vi "Data handler-Motor Zstack.vi"(4 "Save image":bool, 6 "Single Frame Data":T2, 8 "error in (no error)":errorcluster, 9 "Live graph data queue in":T1, 10 "Logging queue element in":T5={"Imaging Protocol"=enum."Live Imaging", "Number of Trials"=0, "Frame Size"=512, "# Averaged frames"=0, "Dwell time (us)"=0.0, "Index of Z-plane"=0, "Timelapse?"=FALSE, "Logging process is active"=FALSE, "Speed logging enabled"=FALSE, "tdms file ref"=refnum, "path"=path "", "Trial Number"=0, "Expected # points acquired"=FALSE, "Manually stopped"=FALSE, "Last trial"=FALSE, "Ch0 data"=[], "Ch1 data"=[], "Image Time"=[], "Continuous Time"=[], "Points acquired"={"Ch0 last trial"=0, "Ch1 last trial"=0, "All trials"=0}, "HW Timings File"=refnum} {"Frame Size" items=["100X100"=100, "128X128"=128, "200X200"=200, "256X256"=256, "512X512"=512, "1024x1024"=1024, "2048x2048"=2048]; "Dwell time (us)" format="%#.6g"}, 11 "Image array":T3) -> (0 "error out":errorcluster)   [LabVIEW 2017]
uses:
  Typedefs/Logging queue element.ctl
  Typedefs/Imaging Protocols enum.ctl
  Typedefs/Frame Size.ctl
  Typedefs/Acquired points count.ctl
  User Interface/Queue/Live graphs queue/Typedefs/Live imaging queue element.ctl
  <vilib>/vision/Image Controls.llb/IMAQ Image.ctl
  Typedefs/Frame data dual cluster.ctl
  User Interface/Typedefs/Live graph data queue ref.ctl
  Typedefs/Top level VI states.ctl
  Typedefs/Subpanel close request.ctl
  Global Variables/General Globals.vi
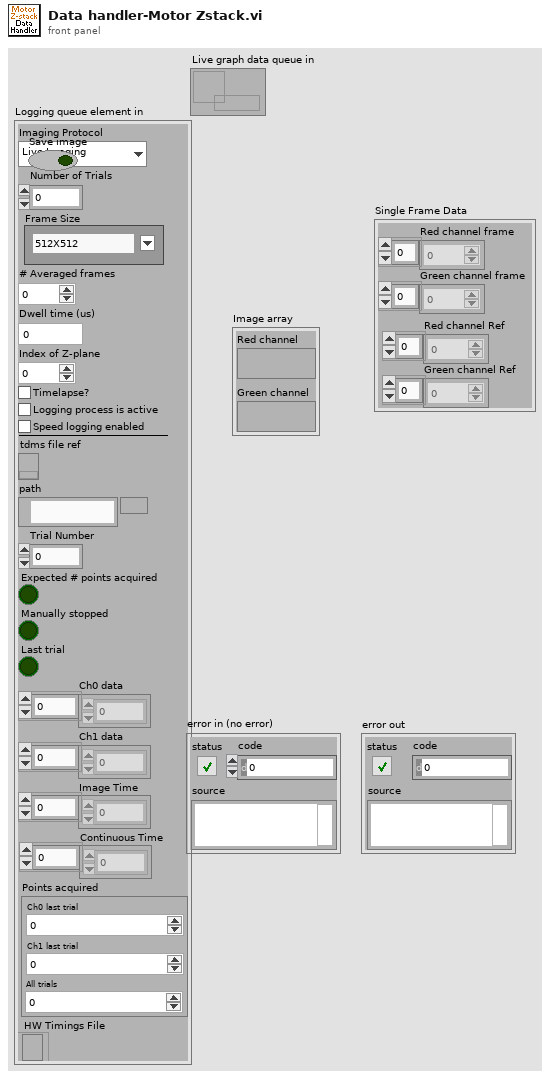
[diagram p1: front panel]
types:
  T1 = typedef "Live graph data queue ref.ctl" = refnum<queue>
  T2 = typedef "Frame data dual cluster.ctl" = cluster{"Red channel frame":dbl[], "Green channel frame":dbl[], "Red channel Ref":dbl[], "Green channel Ref":dbl[]}
  T3 = typedef "Live imaging queue element.ctl" = cluster{"Red channel":T4, "Green channel":T4}
  T4 = typedef "IMAQ Image.ctl" = refnum<image>
  T5 = typedef "Logging queue element.ctl" = cluster{"Imaging Protocol":T6, "Number of Trials":u16, "Frame Size":T7, "# Averaged frames":u16, "Dwell time (us)":dbl, "Index of Z-plane":i32, "Timelapse?":bool, "Logging process is active":bool, "Speed logging enabled":bool, "tdms file ref":refnum<k34>, "path":path, "Trial Number":i32, "Expected # points acquired":bool, "Manually stopped":bool, "Last trial":bool, "Ch0 data":u32[], "Ch1 data":u32[], "Image Time":u64[], "Continuous Time":u64[], "Points acquired":T8, "HW Timings File":refnum<file>}
  T6 = typedef "Imaging Protocols enum.ctl" = enum16{"AOL Z-Stack", "Motor Z Stack", "Functional Acquisition", "Single Plane Acquisition", "Volume Acquisition", "Live Imaging", "Live Plane Imaging", "Live Volume Imaging"}
  T7 = typedef "Frame Size.ctl" = u16
  T8 = typedef "Acquired points count.ctl" = cluster{"Ch0 last trial":u64, "Ch1 last trial":u64, "All trials":u64}
  T9 = typedef "Top level VI states.ctl" = enum16{"None", "Initialise UI", "<STACK PROTOCOL STATES>", "AOL Zstack-START", "AOL Zstack-STOP", "Motor Zstack-START", "Motor Zstack-STOP", "<ACQUISITION PROTOCOL STATES> ", "Functional Acquisition-START", "Functional Acquisition-STOP", "Single Plane Acquisition-START", "Single Plane Acquisition-STOP", "Volume Acquisition-START", "Volume Acquisition-STOP", "<LIVE IMAGING PROTOCOL STATES>", "Live Imaging-START", "Live Imaging-STOP", "Live Plane Imaging-START", "Live Plane Imaging-STOP", "Live Volume Imaging-START", "Live Volume Imaging-STOP", "<MOVEMENT CORRECTION PROTOCOL STATES>", "EXIT"}
  T10 = typedef "Subpanel close request.ctl" = enum16{"Request subpanel close", "Just check subpanel is closed"}
  T11 = enum16{"open", "replace", "create", "open or create", "replace or create", "replace or create with confirmation"}
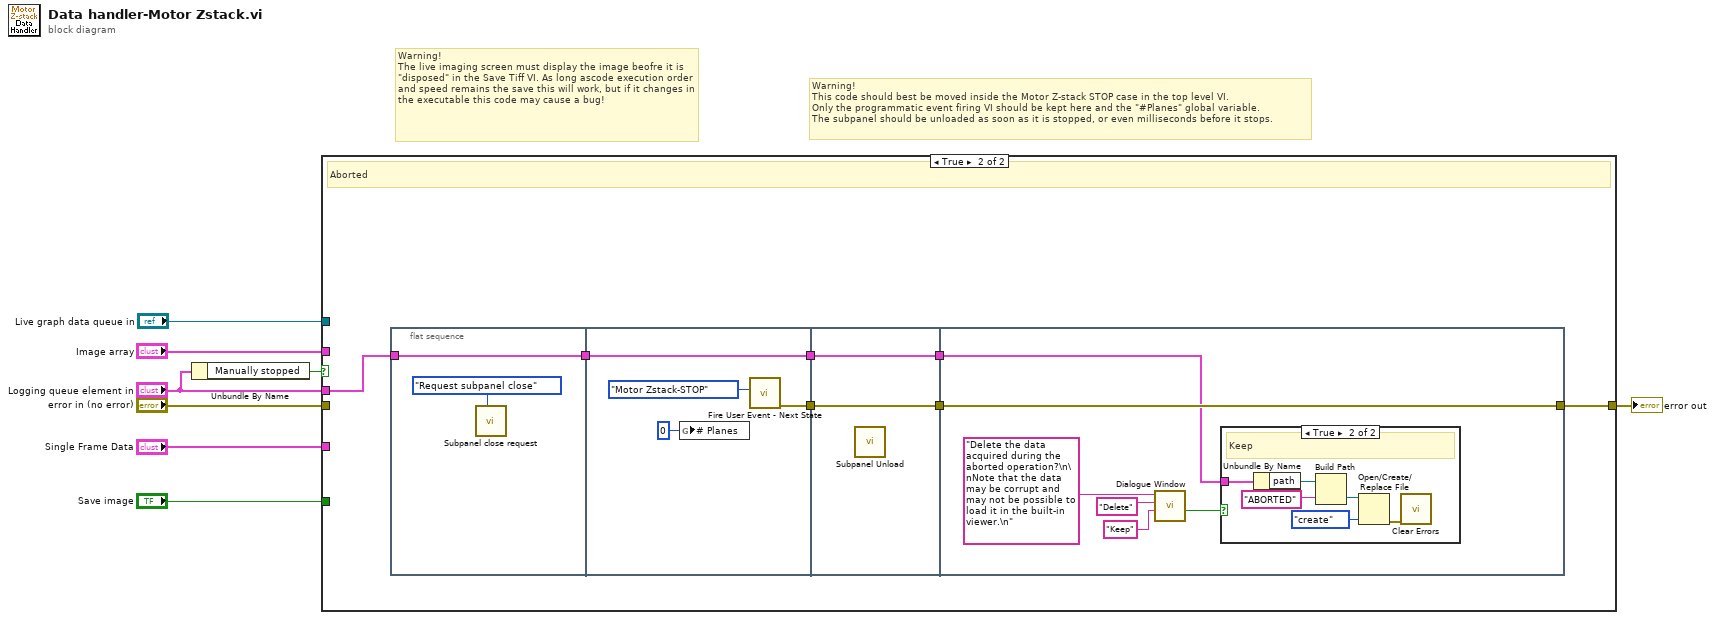
[diagram p0: block diagram]
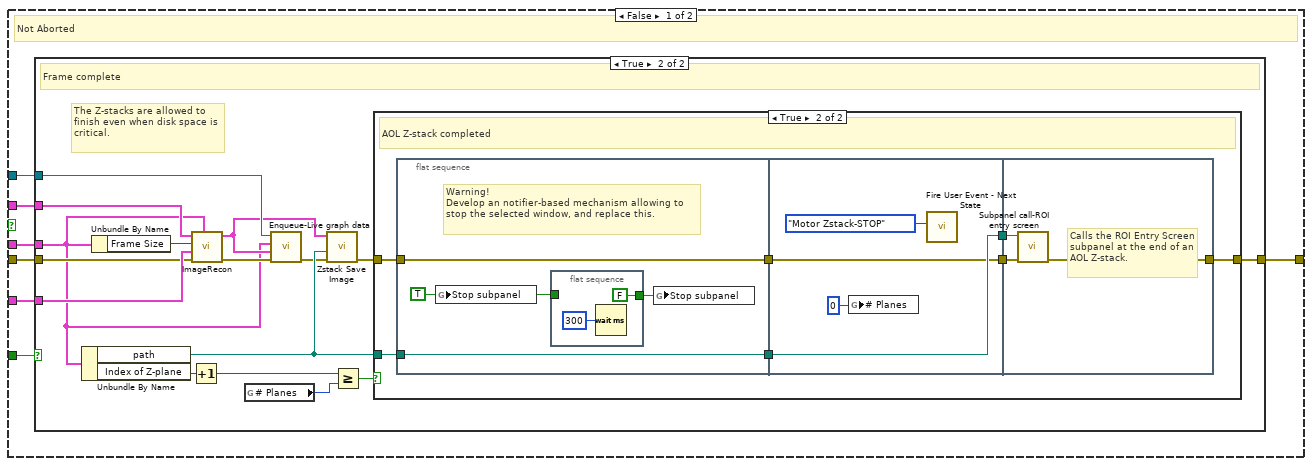
[diagram p2: hidden frame]
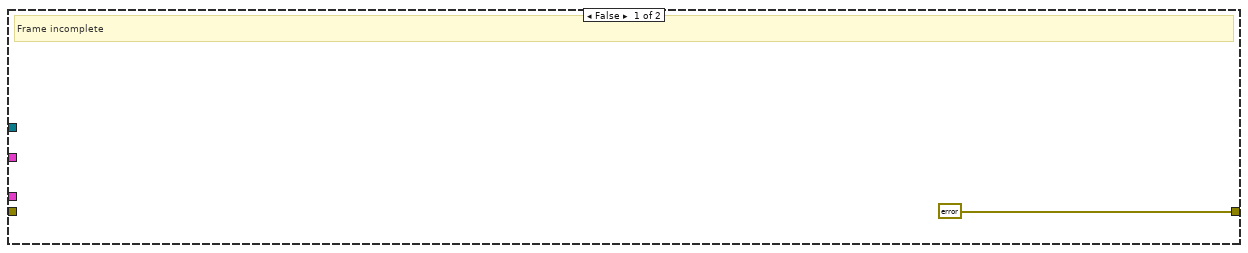
[diagram p3: hidden frame]
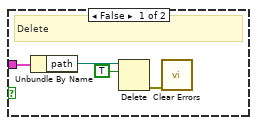
[diagram p5: hidden frame]
diagram:
  # "Warning!\nThe live imaging screen must display the image beofre it is \"disposed\" in the Save Tiff VI. As long ascode execution order and speed remains the save this will work, but if it changes in the executable this code may cause a bug!"
  # "Warning!\nThis code should best be moved inside the Motor Z-stack STOP case in the top level VI.\nOnly the programmatic event firing VI should be kept here and the \"#Planes\" global variable.\nThe subpanel should be unloaded as soon as it is stopped, or even milliseconds before it stops."
  n1 = Unbundle By Name("Logging queue element in") -> ("Manually stopped"=w1:bool)
  n2 = case shown="True" w1 {
    tunnel: [w15 w59] -> w8
    tunnel: "Logging queue element in" -> [w14 w54]
    tunnel: "Image array" -> [w13 _]
    tunnel: "Single Frame Data" -> [w12 _]
    tunnel: "Save image" -> [w11 _]
    tunnel: "error in (no error)" -> [w10 _]
    tunnel: "Live graph data queue in" -> [w9 _]
    frame False {
      # "Not Aborted"
      n3 = case shown="True" w11 {
        tunnel: [errorcluster {"status"=FALSE, "code"=0, "source"=""} ("error out") w32] -> w15
        tunnel: w14 -> [_ w17]
        tunnel: w13 -> [_ w24]
        tunnel: w12 -> [_ w26]
        tunnel: w10 -> [_ w25]
        tunnel: w9 -> [_ w23]
        frame False {
          # "Frame incomplete"
        }
        frame True {
          # "The Z-stacks are allowed to finish even when disk space is critical."
          # "Frame complete"
          n4 = Unbundle By Name(w17) -> ("path"=w27:path, "Index of Z-plane"=w29:i32)
          n5 = Unbundle By Name(w17) -> ("Frame Size"=w30:T7)
          n6 = Increment(x=w29) -> (x+1=w31:i32)
          n7 = call "ImageRecon.vi"("Logging queue element in"=w17, "Error In"=w25, "Data"=w26, "Frame Size"=w30, "Image Array (in)"=w24) -> ("Error Out"=w19:errorcluster, "Image Array(out)"=w22:T3)  [unwired: 3 in, 2 out]
          n8 = global read "General Globals.vi" "# Planes"() -> (w18:i32)
          n9 = call "Enqueue-Live graph data.vi"("error in (no error)"=w19, "Element to queue"=w22, "Logging queue element"=w17, "Live graph data queue in"=w23) -> ("error out"=w20:errorcluster)  [unwired: 6 in, 1 out]
          n10 = call "Zstack Save Image.vi"("error in (no error)"=w20, "Dataset base-path"=w27, "Image Array"=w22) -> ("error out"=w21:errorcluster)  [unwired: 8 in]
          n11 = Greater Or Equal?(x=w31, y=w18) -> (x >= y?=w28:bool)
          n12 = case shown="True" w28 {
            tunnel: w21 -> [w33 w36]
            tunnel: w27 -> [_ w40]
            tunnel: [w33 w39] -> w32
            frame False {
            }
            frame True {
              # "AOL Z-stack completed"
              n13 = flat-sequence {
                tunnel: w36 -> [w43]
                tunnel: w40 -> [w44]
                tunnel: [w44] -> w35
                tunnel: [w43] -> w34
                tunnel: [w50] -> w38
                tunnel: [w48] -> w37
                tunnel: w35 -> [w50]
                tunnel: w34 -> [w48]
                tunnel: [w52] -> w39
                tunnel: w38 -> [w53]
                tunnel: w37 -> [w51]
                frame #0 {
                  w42 = TRUE ("Stop subpanel")
                  # "Warning!\nDevelop an notifier-based mechanism allowing to stop the selected window, and replace this."
                  n14 = global write "General Globals.vi" "Stop subpanel"(w42) -> ()
                  n15 = flat-sequence {
                    tunnel: w42 -> [_]
                    tunnel: [FALSE] -> w41
                    frame #0 {
                      n16 = Wait (ms)(milliseconds to wait=u32 300) -> ()  [unwired: 1 out]
                    }
                  }
                  n17 = global write "General Globals.vi" "Stop subpanel"(w41) -> ()
                }
                frame #1 {
                  n18 = global write "General Globals.vi" "# Planes"(0 ("# Planes")) -> ()
                  n19 = call "Fire User Event - Next State.vi"("\"UI Handler loop\" case to execute"=Top_level_VI_states."Motor Zstack-STOP" ("event data / imaging mode")) -> ()  [unwired: 10 in, 1 out]
                }
                frame #2 {
                  # "Calls the ROI Entry Screen subpanel at the end of an AOL Z-stack."
                  n20 = call "Subpanel call-ROI entry screen.vi"("error in"=w51, "Experiment folder path"=w53) -> ("error out"=w52:errorcluster)  [unwired: 9 in]
                }
              }
            }
          }
        }
      }
    }
    frame True {
      # "Aborted"
      n21 = flat-sequence {
        tunnel: [w61] -> w55
        tunnel: w54 -> [w61]
        tunnel: [w64] -> w60
        tunnel: [w63] -> w56
        tunnel: w55 -> [w63]
        tunnel: w60 -> [w68]
        tunnel: [w68] -> w58
        tunnel: [w67] -> w57
        tunnel: w56 -> [w67]
        tunnel: [w74] -> w59
        tunnel: w58 -> [w74]
        tunnel: w57 -> [w69]
        frame #0 {
          n22 = call "Subpanel close request.vi"("Function"=Subpanel_close_request."Request subpanel close") -> ()  [unwired: 10 in, 1 out]
        }
        frame #1 {
          n23 = global write "General Globals.vi" "# Planes"(0 ("# Planes")) -> ()
          n24 = call "Fire User Event - Next State.vi"("\"UI Handler loop\" case to execute"=Top_level_VI_states."Motor Zstack-STOP" ("event data / imaging mode")) -> ("Error Out"=w64:errorcluster)  [unwired: 10 in]
        }
        frame #2 {
          n25 = call "Subpanel Unload.vi"() -> ()  [unwired: 11 in, 1 out]
        }
        frame #3 {
          n26 = call "Dialogue Window.vi"("Caption-Left button (Cancel)"="Keep", "Caption-Right button (OK)"="Delete", "Message string"="Delete the data acquired during the aborted operation?\n\nNote that the data may be corrupt and may not be possible to load it in the built-in viewer.\n") -> ("Cancelled (Left button pressed)"=w71:bool)  [unwired: 6 in, 2 out]
          n27 = case shown="True" w71 {
            tunnel: w69 -> [w78 w79]
            frame False {
              # "Delete"
              n28 = Unbundle By Name(w78) -> ("path"=w77:path)
              n29 = Delete(path (use dialog)=w77, entire hierarchy (F)=TRUE) -> (error out=w75:errorcluster)  [unwired: 3 in, 2 out]
              n30 = call <vilib>:"Clear Errors.vi"("error in (no error)"=w75) -> ()  [unwired: 5 in, 2 out]
            }
            frame True {
              # "Keep"
              n31 = Unbundle By Name(w79) -> ("path"=w84:path)
              n32 = Build Path(base path=w84, name or relative path="ABORTED") -> (appended path=w81:path)
              n33 = Open/Create/Replace File(file path (use dialog)=w81, operation (0:open)=T11."create") -> (error out=w83:errorcluster)  [unwired: 4 in, 2 out]
              n34 = call <vilib>:"Clear Errors.vi"("error in (no error)"=w83) -> ()  [unwired: 5 in, 2 out]
            }
          }
        }
      }
    }
  }
  "error out" <- w8
